vi "Timing.vi"(9 "Period (ms)":u32, 10 "Speed":u16, 11 "Time Elapsed In (s)":dbl) -> (2 "Time Elapsed Out (s)":dbl, 3 "Time Interval (s)":dbl)   [LabVIEW 2019]
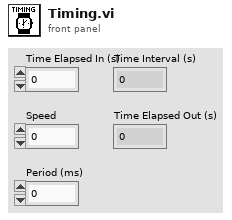
[diagram p1: front panel]
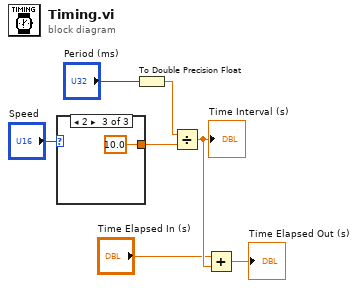
[diagram p0: block diagram]
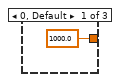
[diagram p2: hidden frame]
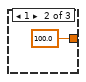
[diagram p3: hidden frame]
diagram:
  n1 = case shown="2" "Speed" {
    tunnel: [1000.0 100.0 ("y") 10.0 ("y")] -> w3
    frame 0, Default {
    }
    frame 1 {
    }
    frame 2 {
    }
  }
  n2 = To Double Precision Float(number="Period (ms)") -> (double precision float=w1:dbl)
  n3 = Divide(x=w1, y=w3) -> (x/y=w7:dbl)
  "Time Interval (s)" <- w7
  n4 = Add(x="Time Elapsed In (s)", y=w7) -> (x+y=→"Time Elapsed Out (s)":dbl)
